vi "Strip Single Control (Variant).vi"(0 "Ctl Refnum":refnum<vi>, 1 "Cluster Refnum":refnum<vi>, 3 "Label.Text":string, 5 "Keys in":string[](array[string]), 7 "Values in":variant[](array[variant]), 11 "error in (no error)":errorcluster, 12 "Strip Cluster":refnum<vi>, 14 "Value":variant) -> (4 "Ctl Refnum":refnum<vi>, 6 "Keys out":string[](array[string]), 8 "Values out":variant[](array[variant]), 15 "error out":errorcluster)   [LabVIEW 2017]
panel:
  in  "type specifier":refnum<vi>
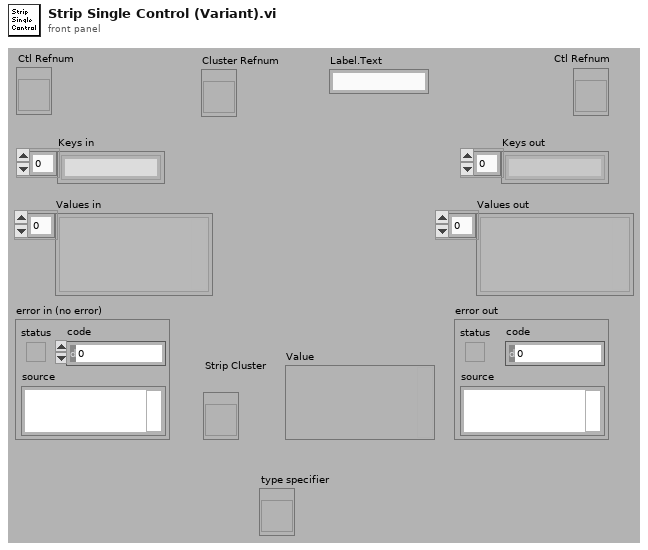
[diagram p1: front panel]
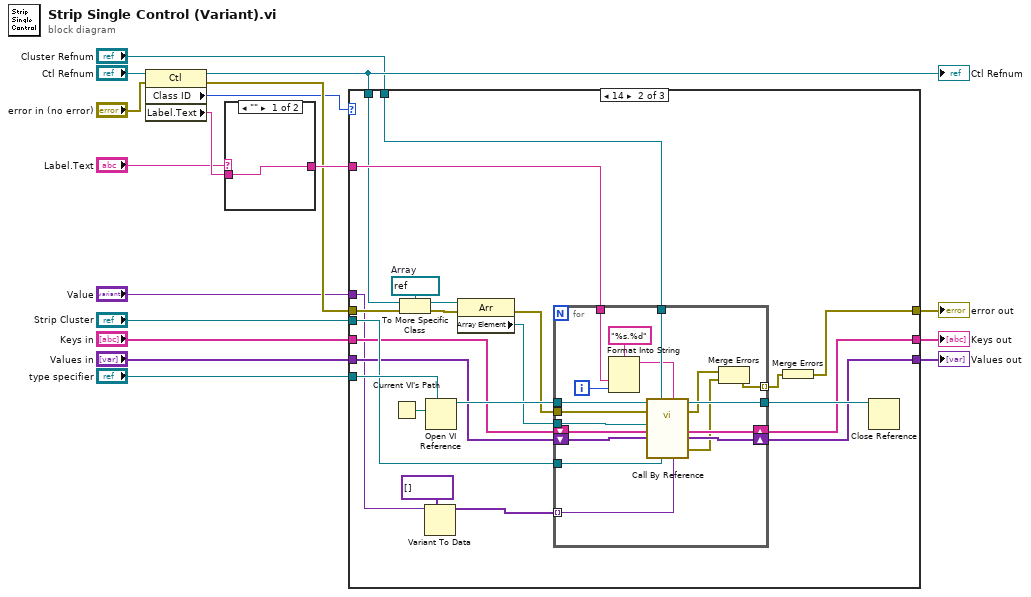
[diagram p0: block diagram]
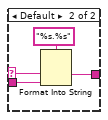
[diagram p2: hidden frame]
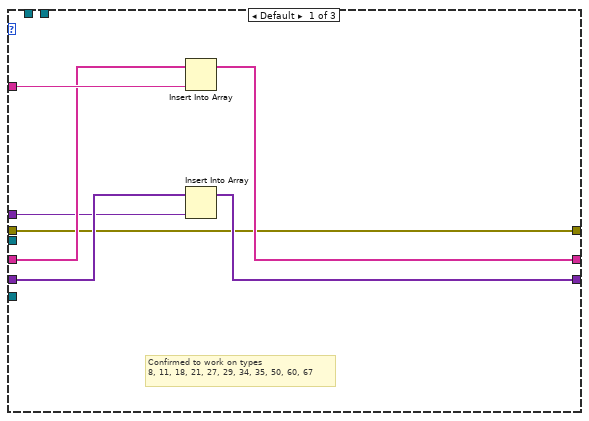
[diagram p3: hidden frame]
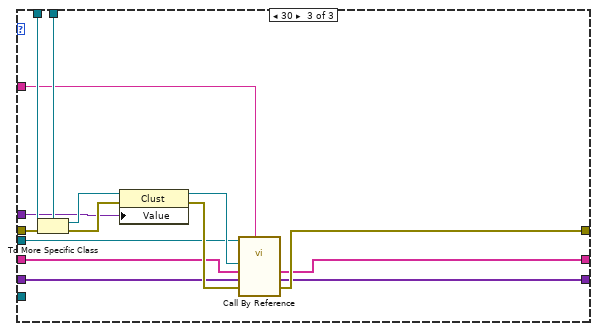
[diagram p4: hidden frame]
diagram:
  n1 = property class="Ctl"(reference="Ctl Refnum", error in="error in (no error)") -> (reference out=w17:refnum<vi>, error out=w8:errorcluster, "Class ID"=w6:u32, "Label.Text"=w16:string)
  "Ctl Refnum" <- w17
  n2 = case shown="\"\"" "Label.Text" {
    selector: "Label.Text" -> [_ w19]
    tunnel: w16 -> [w18 w22]
    tunnel: [w18 w21] -> w11
    frame "" {
    }
    frame Default {
      n3 = Format Into String(format string="%s.%s", w19, w22) -> (resulting string=w21:string)  [unwired: 2 in, 1 out]
    }
  }
  n4 = case shown="14" w6 {
    tunnel: "Value" -> [w24 w30 w80]
    tunnel: w8 -> [w23 w31 w83]
    tunnel: [w23 w33 w74] -> w9
    tunnel: "Strip Cluster" -> [_ w48 w71]
    tunnel: "Cluster Refnum" -> [_ w39 w84]
    tunnel: w11 -> [w29 w35 w75]
    tunnel: [w26 w41 w72] -> w14
    tunnel: "Keys in" -> [w28 w43 w77]
    tunnel: "Values in" -> [w27 w42 w78]
    tunnel: [w25 w40 w73] -> w15
    tunnel: w17 -> [_ w32 w85]
    tunnel: "type specifier" -> [_ w49 _]
    frame Default {
      # "Confirmed to work on types\n8, 11, 18, 21, 27, 29, 34, 35, 50, 60, 67"
      n5 = Insert Into Array(array=w28, new element=w29) -> (w26:string[])  [unwired: 1 in]
      n6 = Insert Into Array(array=w27, new element=w24) -> (w25:variant[])  [unwired: 1 in]
    }
    frame 14 {
      w47 = refnum<vi> refnum  # Array
      n7 = Current VI's Path() -> (path=w52:path)
      n8 = To More Specific Class(target class=w47, reference=w32, error in=w31) -> (specific class reference=w46:refnum<vi>, error out=w45:errorcluster)
      n9 = Variant To Data(type=variant[] [], Variant=w30) -> (data=w37:variant[])  [unwired: 1 in, 1 out]
      n10 = Open VI Reference(type specifier VI Refnum (for type only)=w49, vi path=w52) -> (vi reference=w51:refnum<vi>)  [unwired: 4 in, 1 out]
      n11 = property class="Arr"(reference=w46, error in=w45) -> (error out=w38:errorcluster, "Array Element"=w44:refnum<vi>)  [unwired: 1 out]
      n12 = for {
        tunnel: w51 -> [w70]
        tunnel: [w69] -> w50
        tunnel: w48 -> [w53]
        tunnel: w44 -> [w68]
        tunnel: w39 -> [w63]
        shift-right: [w65] -> w41
        shift-left: w43 -> [w67]
        shift-right: [w64] -> w40
        shift-left: w42 -> [w66]
        tunnel: w38 -> [w62]
        tunnel: w37 -> [w54] mode=indexing
        tunnel: w35 -> [w60]
        tunnel: [w55] -> w34 mode=indexing
        i -> [w59]
        n13 = Format Into String(format string="%s.%d", w60, w59) -> (resulting string=w58:string)  [unwired: 2 in, 1 out]
        n14 = call-by-ref "?"(reference=w70, error in=w62, "Ctl Refnum"=w68, "Cluster Refnum"=w63, "Label.Text"=w58, "Keys in"=w67, "Values in"=w66, "Strip Cluster"=w53, "Value"=w54) -> (reference out=w69:refnum<vi>, error out=w57:errorcluster, "Keys out"=w65:string[], "Values out"=w64:variant[], 15:"error out"=w56:errorcluster)  [unwired: 5 in, 1 out]
        n15 = Merge Errors(w57, w56) -> (w55:errorcluster)
      }
      n16 = Merge Errors(w34) -> (w33:errorcluster)
      n17 = Close Reference(reference=w50) -> ()  [unwired: 1 in, 1 out]
    }
    frame 30 {
      n18 = To More Specific Class(target class=w84, reference=w85, error in=w83) -> (specific class reference=w82:refnum<vi>, error out=w81:errorcluster)
      n19 = property class="Clust"(reference=w82, error in=w81, "Value"=w80) -> (reference out=w76:refnum<vi>, error out=w79:errorcluster)
      n20 = call-by-ref "?"(reference=w71, "Prefix Name"=w75, "error in (no error)"=w79, "Values in"=w78, "Key in"=w77, "Cluster Refnum"=w76) -> ("error out"=w74:errorcluster, "Values"=w73:variant[], "Keys"=w72:string[])  [unwired: 4 in, 3 out]
    }
  }
  "Values out" <- w15
  "Keys out" <- w14
  "error out" <- w9
